vi "Next Runnable in Suite.vi"(8 "error in (no error)":errorcluster, 11 "LUnit Test Suite In":refnum<class "LUnit Test Suite.lvclass">) -> (0 "error out":errorcluster, 2 "Next":string, 3 "LUnit Test Suite Out":refnum<class "LUnit Test Suite.lvclass">)   [LabVIEW 2020, in "LUnit Test Suite.lvclass"]
uses:
  LUnit Test Suite.lvclass
  LUnit Test Suite.lvclass/LUnit Test Suite.ctl
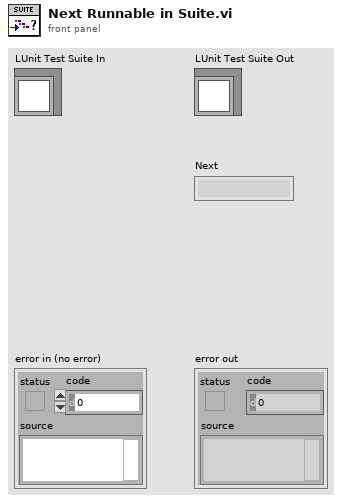
[diagram p1: front panel]
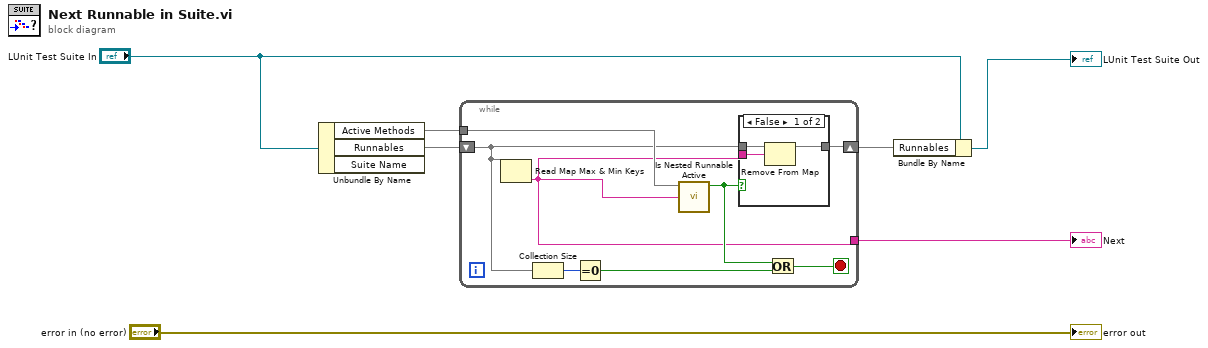
[diagram p0: block diagram]
diagram:
  n1 = Unbundle By Name("LUnit Test Suite In") -> ("Active Methods"=w2:set{string}, "Runnables"=w3:map{string, refnum<class "Runnable.lvclass">})  [unwired: 1 out]
  n2 = while {
    tunnel: w2 -> [w15]
    shift-right: [w14] -> w1
    shift-left: w3 -> [w9]
    tunnel: [w8] -> w5
    stop <- w13 stop-if-true
    n3 = Read Map Max & Min Keys(11:w9) -> (1:w8:string)  [unwired: 1 out]
    n4 = Collection Size(1:w9) -> (0:w12:i32)
    n5 = Equal To 0?(x=w12) -> (x = 0?=w11:bool)
    n6 = call "Is Nested Runnable Active"("Name"=w8, "Active Methods"=w15) -> ("found?"=w10:bool)  [unwired: 9 in]
    n7 = case shown="False" w10 {
      tunnel: w8 -> [w18 _]
      tunnel: [w17 w19] -> w14
      tunnel: w9 -> [w16 w19]
      frame False {
        n8 = Remove From Map(10:w18, 11:w16) -> (3:w17:map{string, refnum<class "Runnable.lvclass">})  [unwired: 2 out]
      }
      frame True {
      }
    }
    n9 = Or(x=w10, y=w11) -> (x .or. y?=w13:bool)
  }
  "Next" <- w5
  n10 = Bundle By Name(cluster="LUnit Test Suite In", "Runnables"=w1) -> (→"LUnit Test Suite Out":refnum<class "LUnit Test Suite.lvclass">)
  "error out" <- "error in (no error)"
